vi "More Dialog.vi"(8 "error in (no error)":errorcluster, 10 "State in":T1 caption="State") -> (0 "error out":errorcluster, 1 "Cancelled?":bool, 2 "State out":T1 caption="State")   [LabVIEW 2012, in "ListBox_XControl.xctl"]
doc: "Shows a pop-up display so the user can set the custom properties graphically. \nThis pop-up is found by clicking on the more... entry of the short cut menu."
uses:
  ListBox_XControl.xctl
  Order Type Def.ctl
  ListBox_State.ctl
  Value Filters.ctl
panel:
  in  "Cancel":bool
  in  "OK":bool
  in  "Tab Control":T4(tab)
  in  "Alternating Row Text Color":u32(colorbox)
  in  "Alternating Row Background Color":u32(colorbox)
  in  "Ordering":T2
  in  "Order by Column":i32
  in  "Clear":bool
  in  "Value Filters":T3
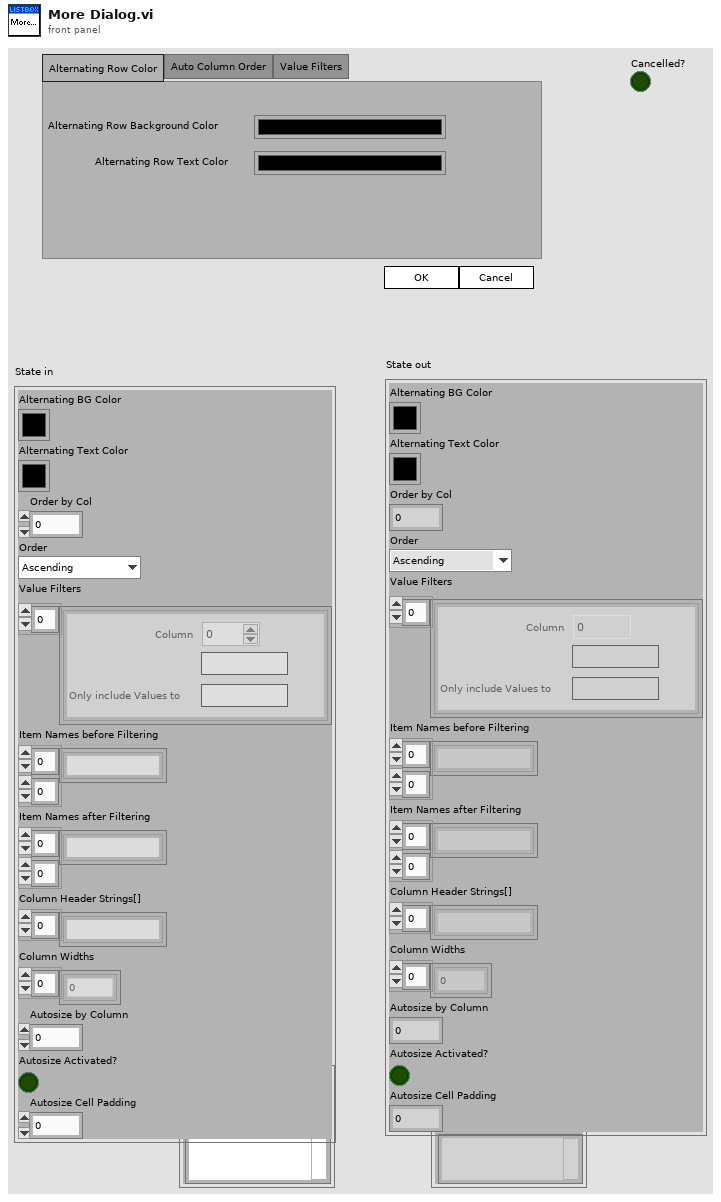
[diagram p1: front panel]
types:
  T1 = typedef "ListBox_XControl.xctl/ListBox_State.ctl" = cluster{"Alternating BG Color":u32, "Alternating Text Color":u32, "Order by Col":i32, "Order":T2, "Value Filters":T3, "Item Names before Filtering":string[][], "Item Names after Filtering":string[][], "Column Header Strings[]":string[], "Column Widths":u32[], "Autosize by Column":i32, "Autosize Activated?":bool, "Autosize Cell Padding":u32}
  T2 = typedef "ListBox_XControl.xctl/Order Type Def.ctl" = enum16{"Ascending", "Descending", "Off"}
  T3 = typedef "ListBox_XControl.xctl/Value Filters.ctl" = cluster{"Column":i32, "Only include Values From":string, "Only include Values to":string}[]
  T4 = enum32{"Alternating Row Color", "Auto Column Order", "Value Filters"}
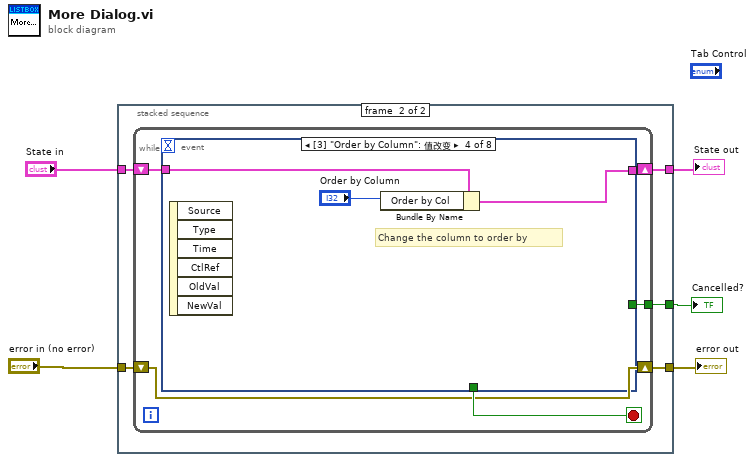
[diagram p0: block diagram]
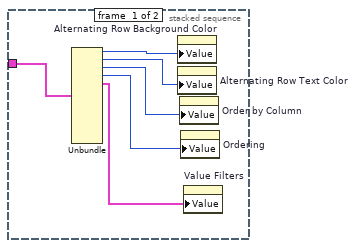
[diagram p2: hidden frame]
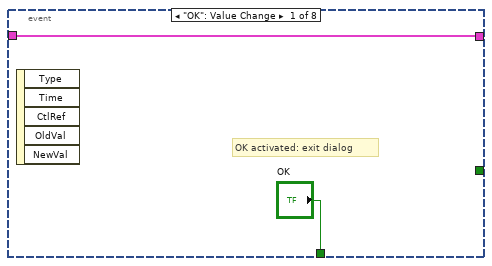
[diagram p3: hidden frame]
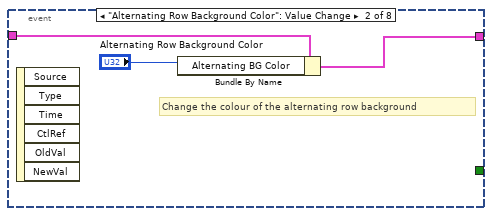
[diagram p4: hidden frame]
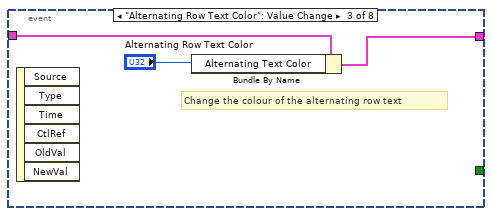
[diagram p5: hidden frame]
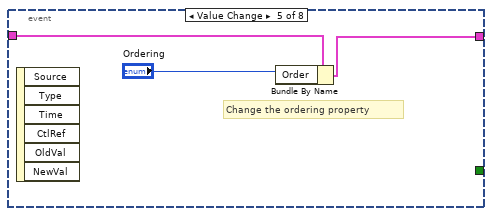
[diagram p6: hidden frame]
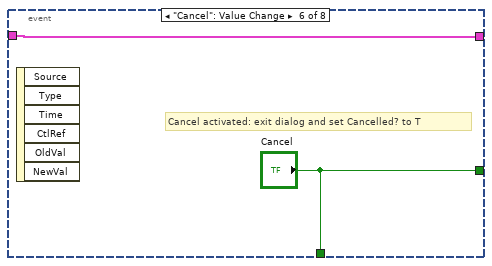
[diagram p7: hidden frame]
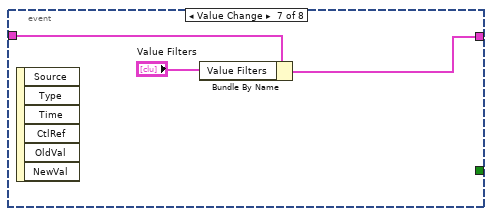
[diagram p8: hidden frame]
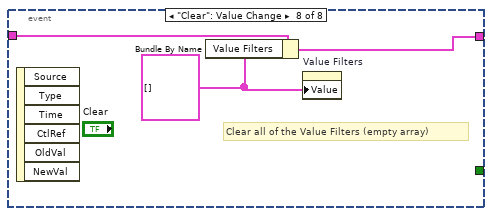
[diagram p9: hidden frame]
diagram:
  n1 = stacked-sequence {
    tunnel: [_ w16] -> w5
    tunnel: "error in (no error)" -> [_ w15]
    tunnel: "State in" -> [w11 w14]
    tunnel: [_ w13] -> w1
    tunnel: [_ w12] -> w3
    frame #0 {
      n2 = Unbundle(w11) -> ("Alternating BG Color"=w10:u32, "Alternating Text Color"=w9:u32, "Order by Col"=w8:i32, "Order"=w7:T2, "Value Filters"=w6:T3)  [unwired: 7 out]
      n3 = property on="Alternating Row Background Color" class="ColBox"("Value"=w10) -> ()  [unwired: 2 in, 2 out]
      n4 = property on="Alternating Row Text Color" class="ColBox"("Value"=w9) -> ()  [unwired: 2 in, 2 out]
      n5 = property on="Order by Column" class="DigNum (严格)"("Value"=w8) -> ()  [unwired: 2 in, 2 out]
      n6 = property on="Ordering" class="Enum (严格)"("Value"=w7) -> ()  [unwired: 2 in, 2 out]
      n7 = property on="Value Filters" class="Arr (严格)"("Value"=w6) -> ()  [unwired: 2 in, 2 out]
    }
    frame #1 {
      n8 = while {
        tunnel: [w20] -> w16
        shift-right: [w17] -> w12
        shift-left: w15 -> [w17]
        shift-right: [w18] -> w13
        shift-left: w14 -> [w19]
        stop <- w21 stop-if-true
        n9 = event shown="[3] \"Order by Column\": 值改变" {
          selector: _ -> [_ _ _ _ _ _ _ _]
          dyn-events: _ -> [_ _ _ _ _ _ _ _]
          timeout: _ -> [_ _ _ _ _ _ _ _]
          tunnel: ["OK" _ _ _ _ "Cancel" _ _] -> w21
          tunnel: [_ _ _ _ _ "Cancel" _ _] -> w20
          tunnel: w19 -> [w22 w26 w29 w32 w34 w36 w40 w43]
          tunnel: [w22 w25 w27 w30 w33 w36 w39 w42] -> w18
          event "OK": Value Change {
            # "OK activated: exit dialog"
            n10 = event-data() -> ()  [unwired: 1 in, 5 out]
          }
          event "Alternating Row Background Color": Value Change {
            # "Change the colour of the alternating row background"
            n11 = event-data() -> ()  [unwired: 1 in, 6 out]
            n12 = Bundle By Name(cluster=w26, "Alternating BG Color"="Alternating Row Background Color") -> (w25:T1)
          }
          event "Alternating Row Text Color": Value Change {
            # "Change the colour of the alternating row text"
            n13 = event-data() -> ()  [unwired: 1 in, 6 out]
            n14 = Bundle By Name(cluster=w29, "Alternating Text Color"="Alternating Row Text Color") -> (w27:T1)
          }
          event "Order by Column": Value Change {
            # "Change the column to order by"
            n15 = event-data() -> ()  [unwired: 1 in, 6 out]
            n16 = Bundle By Name(cluster=w32, "Order by Col"="Order by Column") -> (w30:T1)
          }
          event Value Change {
            # "Change the ordering property"
            n17 = event-data() -> ()  [unwired: 1 in, 6 out]
            n18 = Bundle By Name(cluster=w34, "Order"="Ordering") -> (w33:T1)
          }
          event "Cancel": Value Change {
            # "Cancel activated: exit dialog and set Cancelled? to T"
            n19 = event-data() -> ()  [unwired: 1 in, 6 out]
          }
          event Value Change {
            n20 = event-data() -> ()  [unwired: 1 in, 6 out]
            n21 = Bundle By Name(cluster=w40, "Value Filters"="Value Filters") -> (w39:T1)
          }
          event "Clear": Value Change {
            w41 = T3 [] ("Value Filters")
            # "Clear all of the Value Filters (empty array)"
            n22 = event-data() -> ()  [unwired: 1 in, 6 out]
            n23 = Bundle By Name(cluster=w43, "Value Filters"=w41) -> (w42:T1)
            n24 = property on="Value Filters" class="Arr (严格)"("Value"=w41) -> ()  [unwired: 2 in, 2 out]
          }
        }
      }
    }
  }
  "Cancelled?" <- w5
  "error out" <- w3
  "State out" <- w1
